vi "sample obtain and delete object.vi"() -> ()   [LabVIEW 2015]
uses:
  Core/HTTP Request/AWS Credentials.ctl
  Bucket/Bucket.lvclass
  Core/HTTP Request/HTTP Request.lvclass
panel:
  in  "Object Key":string
  out "error out":errorcluster
  in  "Bucket name":string="bpreis-test-95"
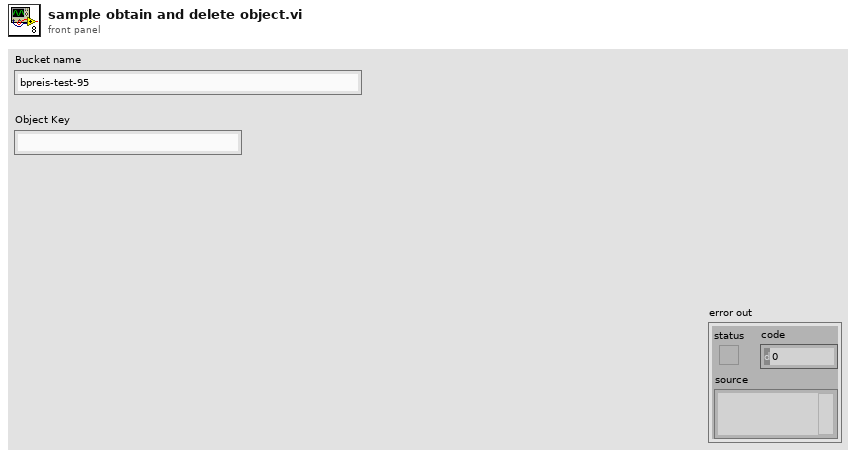
[diagram p1: front panel]
types:
  T1 = typedef "NI_AWS_Core.lvlib/HTTP Request.lvclass/AWS Credentials.ctl" = cluster{"Access Key":string, "Secret Key":string}
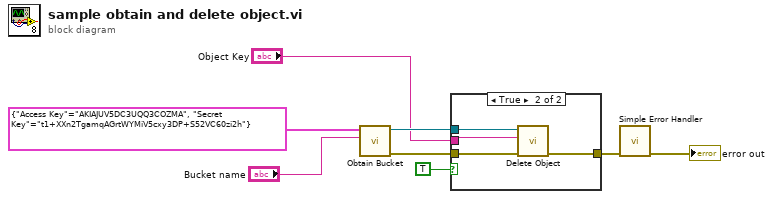
[diagram p0: block diagram]
diagram:
  n1 = call "Obtain Bucket.vi"("Bucket name"="Bucket name", "AWS Credentials"=T1 {"Access Key"="AKIAJUV5DC3UQQ3COZMA", "Secret Key"="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"}) -> ("error out"=w8:errorcluster, "Bucket"=w2:refnum<class "Bucket.lvclass">)  [unwired: 8 in]
  n2 = case shown="True" TRUE {
    tunnel: [w9 w13] -> w7
    tunnel: w8 -> [w9 w12]
    tunnel: w2 -> [_ w11]
    tunnel: "Object Key" -> [_ w10]
    frame False {
    }
    frame True {
      n3 = call "Delete Object.vi"("error in (no error)"=w12, "Object Key"=w10, "Bucket in"=w11) -> ("error out"=w13:errorcluster)  [unwired: 7 in, 1 out]
    }
  }
  n4 = call <vilib>:"Simple Error Handler.vi"("error in (no error)"=w7) -> ("error out"=→"error out":errorcluster)  [unwired: 4 in, 4 out]
